vi "InsertHorizontalLine.vi"(8 "error in (no error)":errorcluster, 10 "ParentTag":string, 11 "MenuStrip in":refnum<class "MGI_MenuStrip.lvclass">) -> (0 "error out":errorcluster, 3 "MenuStrip out":refnum<class "MGI_MenuStrip.lvclass">)   [LabVIEW 2016, in "MGI_MenuStrip.lvclass"]
doc: "Inserts a horizontal line into the menu. Called when a MenuSeparatorItem is added.\n\nAuthored by Derek E. Trepanier\nsupport@mooregoodideas.com\nwww.mooregoodideas.com\n\nCopyright (c) 2012, Moore Good Ideas, Inc.\n\nAll rights reserved.\n\nRedistribution and use in source and binary forms, with or without modification, are permitted provided that the following conditions are met:\n\n * Redistributions of source code must retain the above copyright notice, this list of conditions and the following disclaimer.\n * Redistributions in binary form must reproduce the above copyright notice, this list of conditions and the following disclaimer in the documentation and/or other materials provided with the distribution.\n * Neither the name of Moore Good Ideas, Inc. nor the names of its contributors may be used to endorse or promote products derived from this software without specific prior written permission.\n\nTHIS SOFTWARE IS PROVIDED BY THE COPYRIGHT HOLDERS AND CONTRIBUTORS \"AS IS\" AND ANY EXPRESS OR IMPLIED WARRANTIES, INCLUDING, BUT NOT LIMITED TO, THE IMPLIED WARRANTIES OF MERCHANTABILITY AND FITNESS FOR A PARTICULAR PURPOSE ARE DISCLAIMED. IN NO EVENT SHALL THE COPYRIGHT OWNER OR CONTRIBUTORS BE LIABLE FOR ANY DIRECT, INDIRECT, INCIDENTAL, SPECIAL, EXEMPLARY, OR CONSEQUENTIAL DAMAGES (INCLUDING, BUT NOT LIMITED TO, PROCUREMENT OF SUBSTITUTE GOODS OR SERVICES; LOSS OF USE, DATA, OR PROFITS; OR BUSINESS INTERRUPTION) HOWEVER CAUSED AND ON ANY THEORY OF LIABILITY, WHETHER IN CONTRACT, STRICT LIABILITY, OR TORT (INCLUDING NEGLIGENCE OR OTHERWISE) ARISING IN ANY WAY OUT OF THE USE OF THIS SOFTWARE, EVEN IF ADVISED OF THE POSSIBILITY OF SUCH DAMAGE."
uses:
  <userlib>/_MGI/Menu Building/MenuTypes/MenuStrip/MGI_MenuStrip.lvclass
  <userlib>/_MGI/Menu Building/MenuTypes/MenuStrip/MGI_MenuStrip.lvclass/MGI_MenuStrip.ctl
  System.Windows.Forms
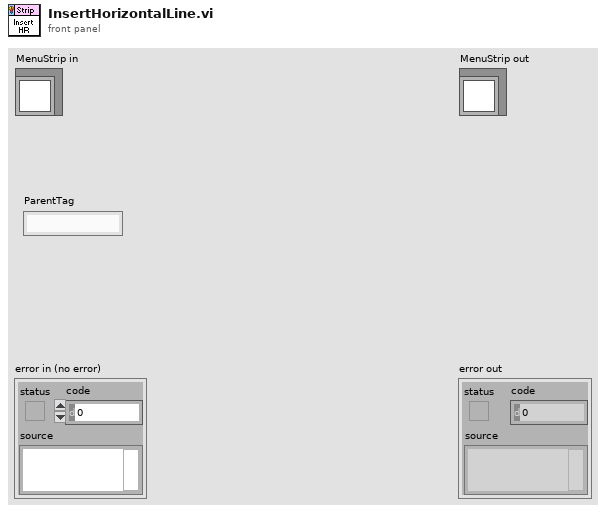
[diagram p1: front panel]
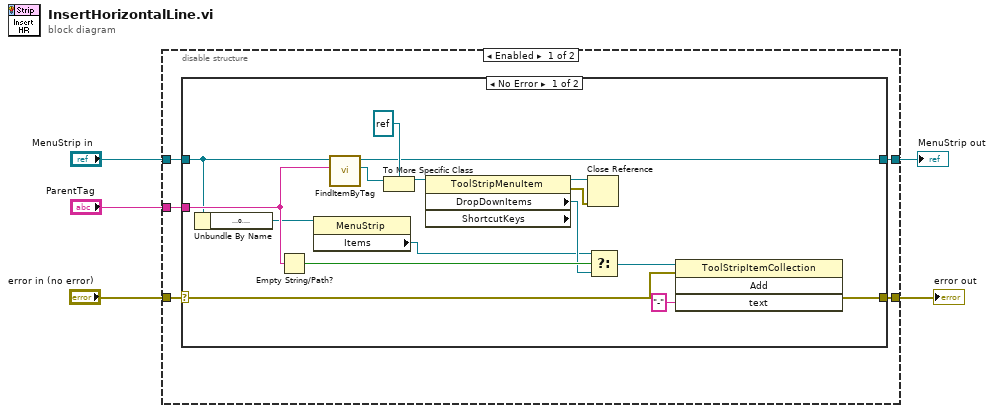
[diagram p0: block diagram]
diagram:
  n1 = disable-structure shown="Enabled" {
    disable-tunnel: "ParentTag" -> [w10 _]
    disable-tunnel: "MenuStrip in" -> [w9 w30]
    disable-tunnel: [w8 w30] -> w3
    disable-tunnel: [w7 w29] -> w2
    disable-tunnel: "error in (no error)" -> [w6 w29]
    frame Enabled {
      n2 = case shown="No Error" w6 {
        selector: w6 -> [w12 w27]
        tunnel: w10 -> [w18 _]
        tunnel: w9 -> [w17 w28]
        tunnel: [w15 w28] -> w8
        tunnel: [w11 w27] -> w7
        frame No Error {
          n3 = Unbundle By Name(w17) -> ("MenuStrip"=w16:refnum<k24>)
          n4 = Empty String/Path?(string/path=w18) -> (empty?=w26:bool)
          n5 = property class="MenuStrip"(reference=w16) -> ("Items"=w21:refnum<k24>)  [unwired: 1 in, 2 out]
          n6 = call <userlib>:"FindItemByTag.vi"("Tag"=w18, "MenuStrip in"=w17) -> ("Tool Strip Menu Item"=w24:refnum<k24>, "MenuStrip out"=w15:refnum<class "MGI_MenuStrip.lvclass">)  [unwired: 7 in, 1 out]
          n7 = To More Specific Class(target class=refnum<k24> refnum ("new reference"), reference=w24) -> (specific class reference=w23:refnum<k24>)  [unwired: 1 in, 1 out]
          n8 = property class="ToolStripMenuItem" props=["DropDownItems", "ShortcutKeys"](reference=w23) -> (reference out=w19:refnum<k24>, error out=w20:errorcluster, "DropDownItems"=w22:refnum<k24>)  [unwired: 1 in, 1 out]
          n9 = Close Reference(reference=w19, error in (no error)=w20) -> ()  [unwired: 1 out]
          n10 = Select(t=w21, s=w26, f=w22) -> (s? t:f=w14:refnum<k24>)
          n11 = invoke class="ToolStripItemCollection" method="Add"(reference=w14, error in=w12, "text"="-") -> (error out=w11:errorcluster)  [unwired: 1 in, 3 out]
        }
        frame Error {
        }
      }
    }
    frame Disabled {
    }
  }
  "error out" <- w2
  "MenuStrip out" <- w3
